vi "ManipSetRobotPosition.vi"(2 "Reinit":bool, 3 "Parameter String":string) -> (0 "Error Out":errorcluster, 1 "Advance Trigger":bool)   [LabVIEW 2020]
doc: "This VI sets the robot position. This can be used to zero out accumulated position error based on a fiducial. Pass -1 as arguments to re-sync the odometry-only pose with the fused pose estimate.\n\nParameters:\n1. X location --> (in) [-1,field length]\n2. Y location --> (in) [-1,field width]"
uses:
  GlobalPoseAndTargeting.vi
  SafeParser_Float.vi
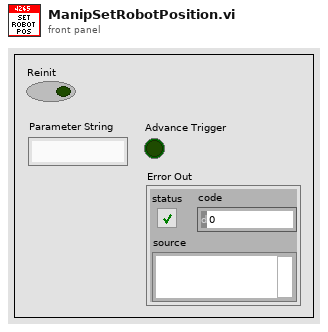
[diagram p1: front panel]
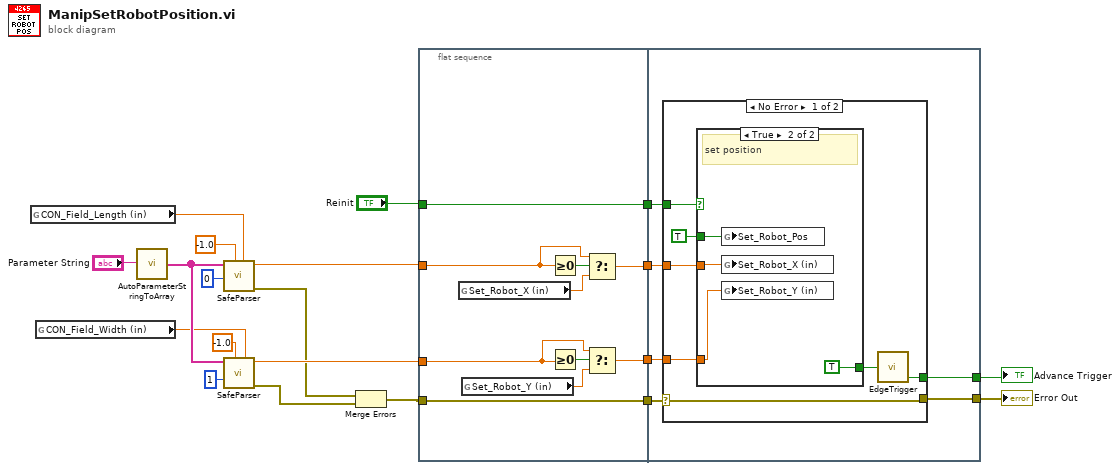
[diagram p0: block diagram]
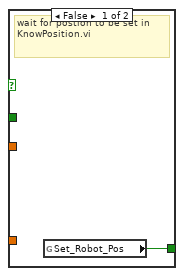
[diagram p2: hidden frame]
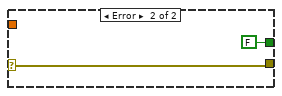
[diagram p3: hidden frame]
diagram:
  n1 = global read "GlobalPoseAndTargeting.vi" "CON_Field_Length (in)"() -> (w2:dbl)
  n2 = global read "GlobalPoseAndTargeting.vi" "CON_Field_Width (in)"() -> (w1:dbl)
  n3 = call "AutoParameterStringToArray.vi"("Parameter String"="Parameter String") -> ("Parsed Parameters"=w15:string[])
  n4 = call-poly "SafeParser.vi"("Maximum"=w2, "Minimum"=-1.0, "Array Index"=0 ("Parameter Index"), "String Array"=w15) -> ("Error Out"=w9:errorcluster, "Typecast  Value"=w11:dbl)  [unwired: 6 in]
  n5 = call-poly "SafeParser.vi"("Maximum"=w1, "Minimum"=-1.0, "Array Index"=1 ("Parameter Index"), "String Array"=w15) -> ("Error Out"=w12:errorcluster, "Typecast  Value"=w10:dbl)  [unwired: 6 in]
  n6 = Merge Errors(w9, w12) -> (w13:errorcluster)
  n7 = flat-sequence {
    tunnel: w10 -> [w24]
    tunnel: w11 -> [w27]
    tunnel: w13 -> [w29]
    tunnel: "Reinit" -> [w30]
    tunnel: [w30] -> w6
    tunnel: [w29] -> w5
    tunnel: [w26] -> w4
    tunnel: [w23] -> w3
    tunnel: [w35] -> w19
    tunnel: [w34] -> w18
    tunnel: w6 -> [w36]
    tunnel: w5 -> [w33]
    tunnel: w4 -> [w32]
    tunnel: w3 -> [w31]
    frame #0 {
      n8 = global read "GlobalPoseAndTargeting.vi" "Set_Robot_X (in)"() -> (w22:dbl)
      n9 = global read "GlobalPoseAndTargeting.vi" "Set_Robot_Y (in)"() -> (w21:dbl)
      n10 = Greater Or Equal To 0?(x=w27) -> (x >= 0?=w28:bool)
      n11 = Greater Or Equal To 0?(x=w24) -> (x >= 0?=w25:bool)
      n12 = Select(t=w27, s=w28, f=w22) -> (s? t:f=w26:dbl)
      n13 = Select(t=w24, s=w25, f=w21) -> (s? t:f=w23:dbl)
    }
    frame #1 {
      n14 = case shown="No Error" w33 {
        selector: w33 -> [w38 w50]
        tunnel: w36 -> [w43 _]
        tunnel: w32 -> [w42 _]
        tunnel: [w39 FALSE ("Falling Edge Trigger")] -> w35
        tunnel: [w38 w50] -> w34
        tunnel: w31 -> [w37 _]
        frame No Error {
          n15 = case shown="True" w43 {
            tunnel: w42 -> [_ w48]
            tunnel: [w44 TRUE ("Falling Edge Trigger")] -> w40
            tunnel: TRUE -> [_ w46]
            tunnel: w37 -> [_ w45]
            frame False {
              # "wait for postion to be set in KnowPosition.vi"
              n16 = global read "GlobalPoseAndTargeting.vi" "Set_Robot_Pos"() -> (w44:bool)
            }
            frame True {
              # "set position"
              n17 = global write "GlobalPoseAndTargeting.vi" "Set_Robot_Pos"(w46) -> ()
              n18 = global write "GlobalPoseAndTargeting.vi" "Set_Robot_X (in)"(w48) -> ()
              n19 = global write "GlobalPoseAndTargeting.vi" "Set_Robot_Y (in)"(w45) -> ()
            }
          }
          n20 = call "EdgeTrigger.vi"("Input Signal"=w40) -> ("Falling Edge Trigger"=w39:bool)  [unwired: 2 out]
        }
        frame Error {
        }
      }
    }
  }
  "Advance Trigger" <- w19
  "Error Out" <- w18
